vi "SetParam.vi"(8 "error in (no error)":errorcluster caption="entrée d'erreur (pas d'erreur)", 10 "euclidean_distances":T1, 11 "Euclidean_distances.lvclass":refnum<class "Euclidean_distances.lvclass">) -> (0 "error out":errorcluster caption="sortie d'erreur", 3 "Euclidean_distances.lvclass":refnum<class "Euclidean_distances.lvclass">)   [LabVIEW 2020, in "Euclidean_distances.lvclass"]
doc: "Set Parameters"
uses:
  Euclidean_distances.lvclass
  Euclidean_distances.lvclass/Euclidean_distances.ctl
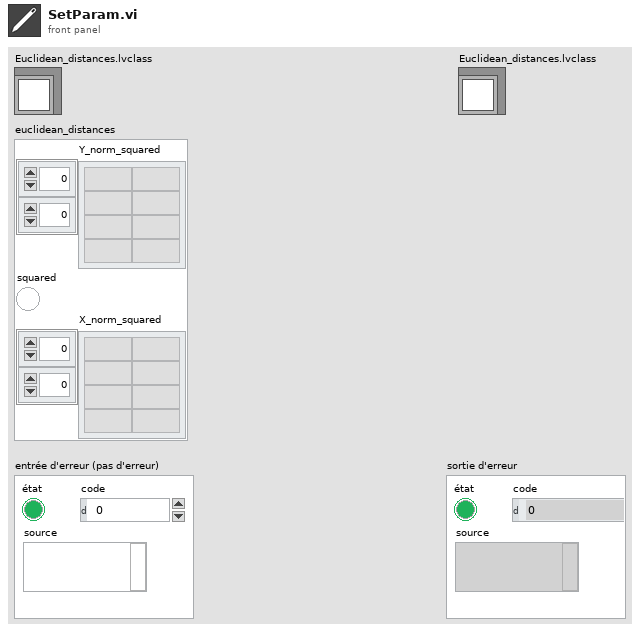
[diagram p1: front panel]
types:
  T1 = cluster{"Y_norm_squared":string[][], "squared":bool, "X_norm_squared":string[][]}
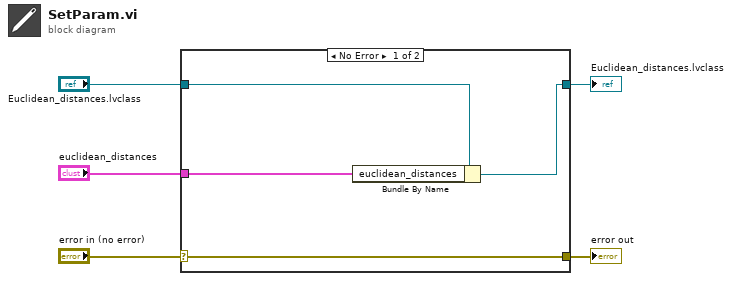
[diagram p0: block diagram]
diagram:
  n1 = case shown="No Error" "error in (no error)" {
    selector: "error in (no error)" -> [w9 w10]
    tunnel: [w9 w10] -> w4
    tunnel: [w7 w11] -> w2
    tunnel: "Euclidean_distances.lvclass" -> [w8 w11]
    tunnel: "euclidean_distances" -> [w6 _]
    frame No Error {
      n2 = Bundle By Name(cluster=w8, "euclidean_distances"=w6) -> (w7:refnum<class "Euclidean_distances.lvclass">)
    }
    frame Error {
    }
  }
  "error out" <- w4
  "Euclidean_distances.lvclass" <- w2
